vi "continuous-serial-read.vi"() -> ()   [LabVIEW 2021]
uses:
  <vilib>/Instr/_visa.llb/VISA Configure Serial Port (Instr).vi
panel:
  in  "index":i32
  out "number":i32
  out "element":string
  out "string array":string[](array[string])
  out "token string":string
  out "string out":string
  in  "Stop Button":bool
  out "Response":string
  out "read buffer":string
  out "return count":u32
  in  "VISA resource name":refnum<visa-resource-name>="COM22"
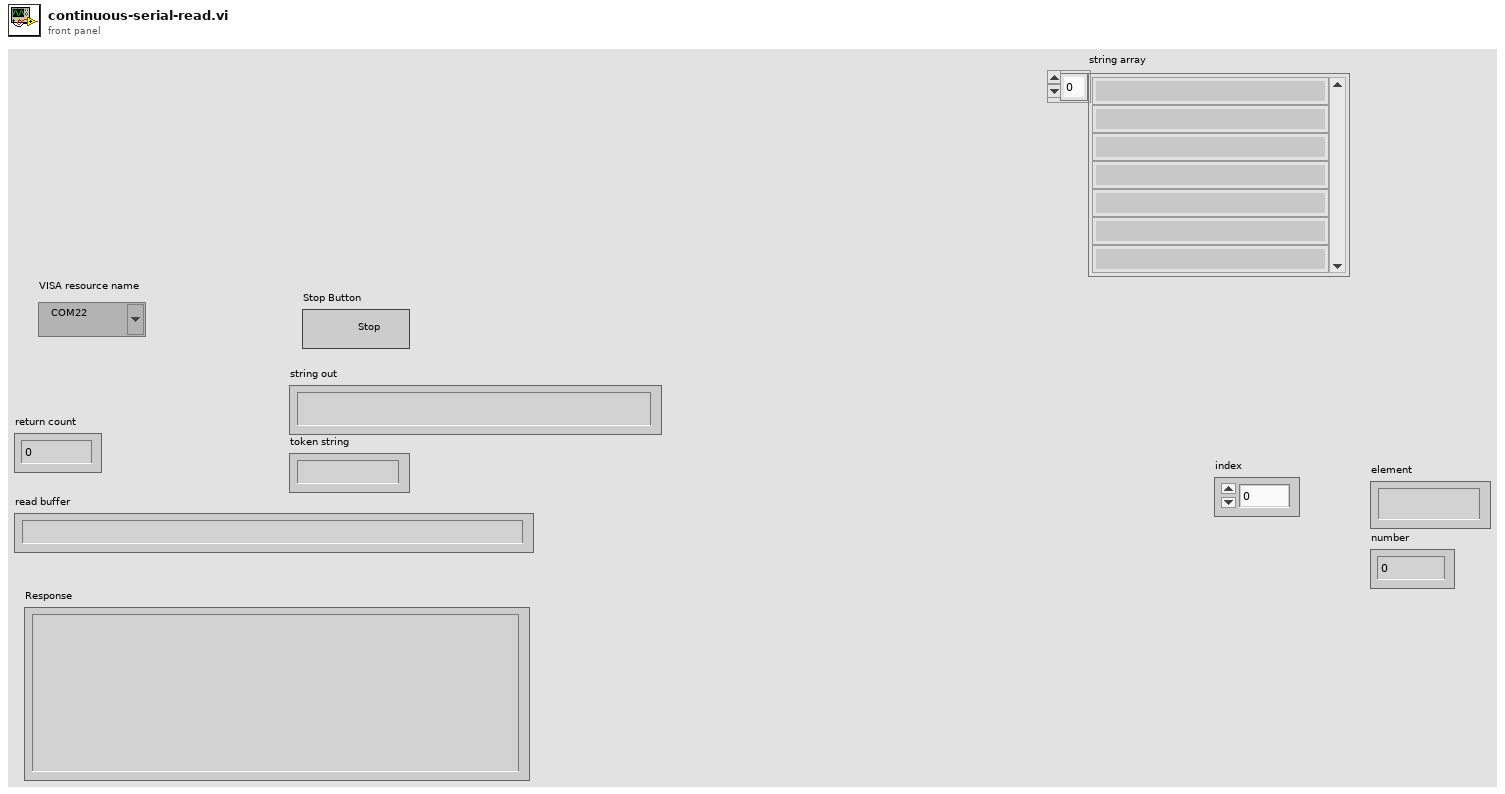
[diagram p1: front panel]
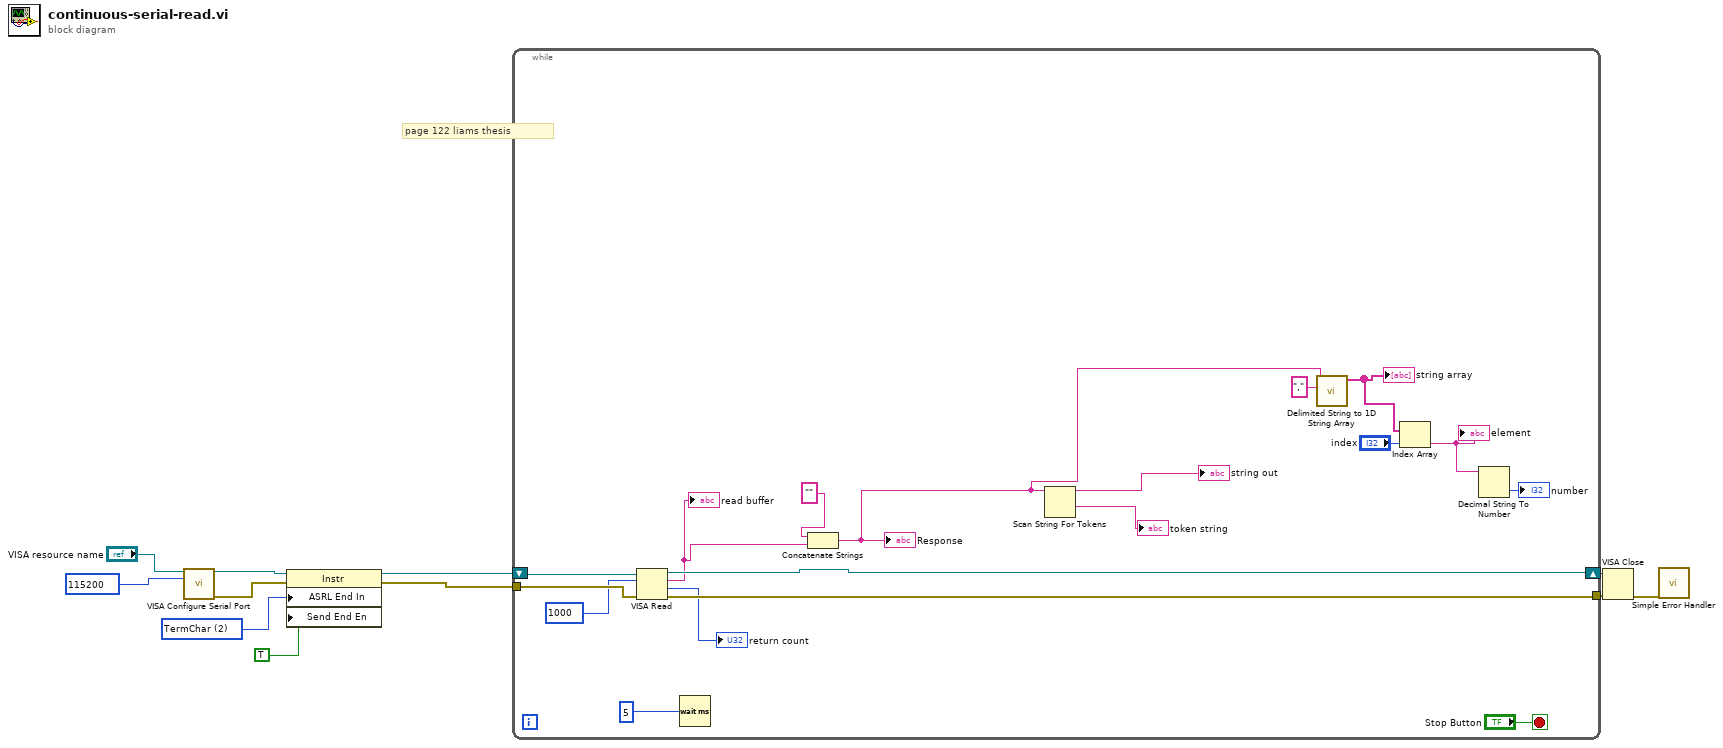
[diagram p0: block diagram]
diagram:
  w7 = u16 2 items=["None", "Last Bit", "TermChar"] ("Serial Settings:End Mode for Reads")
  # "page 122 liams thesis"
  n1 = call-poly "VISA Configure Serial Port"("VISA resource name"="VISA resource name", "baud rate (9600)"=u32 115200) -> ("VISA resource name out"=w9:refnum<visa-resource-name>, "error out"=w8:errorcluster)  [unwired: 12 in]
  n2 = property class="Instr"(reference=w9, error in=w8, "ASRL End In"=w7, "Send End En"=TRUE ("Message Based Settings:Send End Enable")) -> (reference out=w5:refnum<visa-resource-name>, error out=w4:errorcluster)
  n3 = while {
    tunnel: w4 -> [w27]
    shift-right: [w24] -> w2
    shift-left: w5 -> [w29]
    tunnel: [w25] -> w3
    stop <- "Stop Button" stop-if-true
    n4 = VISA Read(VISA resource name=w29, byte count=u32 1000, error in (no error)=w27) -> (VISA resource name out=w24:refnum<visa-resource-name>, read buffer=w20:string, return count=→"return count":u32, error out=w25:errorcluster)
    "read buffer" <- w20
    n5 = Wait (ms)(milliseconds to wait=u32 5) -> ()  [unwired: 1 out]
    n6 = Concatenate Strings("", w20) -> (w16:string)
    "Response" <- w16
    n7 = Scan String For Tokens(9:w16) -> (1:→"token string":string, 3:→"string out":string)  [unwired: 5 in, 2 out]
    n8 = call <vilib>:"Delimited String to 1D String Array.vi"("delimiter"=",", "delimited string"=w16) -> ("string array"=w15:string[])  [unwired: 9 in]
    "string array" <- w15
    n9 = Index Array(array=w15, index="index") -> (element=w14:string)
    "element" <- w14
    n10 = Decimal String To Number(string=w14) -> (number=→"number":i32)  [unwired: 2 in, 1 out]
  }
  n11 = VISA Close(VISA resource name=w2, error in (no error)=w3) -> (error out=w1:errorcluster)
  n12 = call <vilib>:"Simple Error Handler.vi"("error in (no error)"=w1) -> ()  [unwired: 4 in, 5 out]
